vi "PrefDialog.vi"(8 "error in (no error)":errorcluster, 11 "MyPluginsBase in":refnum<class "ChromaAcLoad.lvclass">) -> (0 "error out":errorcluster, 1 "Save As":bool, 2 "Changed":bool, 3 "MyPluginsBase out":refnum<class "ChromaAcLoad.lvclass">)   [LabVIEW 2018, in "AcPwrPlugins.lvlib" / "ChromaAcLoad.lvclass"]
doc: "This VI opens up the modal preference dialog window and allows a user to configure the dialog with a new configuration or the existing configuration that was previously saved to file. The user can also chose to save the new configuration to the existing file location with the save boolean or a new file location by using the save as boolean."
uses:
  ChromaAcLoad.lvclass
  C:/Program Files (x86)/National Instruments/LabVIEW 2018/user.lib/NIST/BaseClasses/BasePlugin_class/BasePlugin.lvclass
  C:/Projects/ICDAS - Local tetsing/NistPluggableModules/AcPwr/AcPwrPlugins/AcPwrBaseClass/AcPwrBase.lvclass
  TypeDefs/Device(s)Settings.ctl
  TypeDefs/ConfigMode.ctl
  AcPwrBaseClass/TypeDefs/BaseMeasurements.ctl
  TypeDefs/MeasurementType.ctl
  TypeDefs/Measurements.ctl
  <userlib>/NIST/BaseClasses/BasePlugin_class/BasePlugin.lvclass/BasePlugin.ctl
  AcPwrBaseClass/AcPwrBase.lvclass/AcPwrBase.ctl
  <userlib>/NIST/BaseClasses/BasePlugin_class/Accessors/Read PluginIniFilePath.vi
  AcPwrBaseClass/Accessors/Read BaseConfig.vi
  AcPwrBaseClass/Accessors/Read BaseMeasurements.vi
  <userlib>/NIST/BaseClasses/BasePlugin_class/Accessors/Write PluginIniFilePath.vi
  <vilib>/Utility/config.llb/NI_LVConfig.lvlib
  AcPwrBaseClass/AcPwrBase.lvclass
panel:
  in  "Measurements":T1 caption="Measurements*"
  in  "BaseMeasurements":T3 {"NHRGridSim Phase" items=["All", "A Phase", "B Phase", "C Phase"]; "NHRDC Measurement Type" items=["Voltage"=1, "Positive Peak Voltage"=2, "Positive Peak Voltage Last Fetch"=4, "Negative Peak Voltage"=8, "Negative Peak Voltage Last Fetch"=16, "Current"=32, "Positive Peak Current"=64, "Positive Peak Current Last Fetch"=128, "Negative Peak Current"=256, "Negative Peak Current Last Fetch"=512, "Power"=1024, "Positive Peak Power"=2048, "Positive Peak Power Last Fetch"=4096, "Negative Peak Power"=8192, "Negative Peak Power Last Fetch"=16384, "Timestamp"=32768, "Charge Time"=65536, "Discharge Time"=131072, "Amp Hour"=262144, "Amp Hour Time"=524288, "Amp Hour Charge"=1048576, "Amp Hour Discharge"=2097152, "Kilo Watt Hour"=4194304, "Kilo Watt Hour Time"=8388608, "Kilo Watt Hour Charge"=16777216, "Kilo Watt Hour Discharge"=33554432, "UUT Temperature"=67108864]; "NHRDC Fetch Method" items=["Aperture", "Immediate"]}
  in  "Disable Controls based on Configuration Mode?":bool
  in  "Device(s)Settings":T4 {"Phases"."Phase Select" items=["Phase ALL", "Phase A", "Phase B", "Phase C"]; "Phases"."Slew Rate"."Fall Slew Rate (A/ms)" min=4 max=600 step=1; "Phases"."Slew Rate"."Rise Slew Rate (A/ms)" min=4 max=600 step=1}
  in  "btnSaveAs":bool
  in  "Measurement RefreshTime (ms)":u32
  in  "btnSave":bool
  in  "btnCancel":bool
  # "*Please ensure that Voltage and Current are selected as the 1st and 2nd Measurement variables, respectively, to correctly plot Voltage vs Current in the visualization VI."
  # "AC is compatible with: CC, CR, CP, RLC, RLC CP, and Inrush\n\nDC is compatible with: CC, CR, CP, CV, and Rectified"
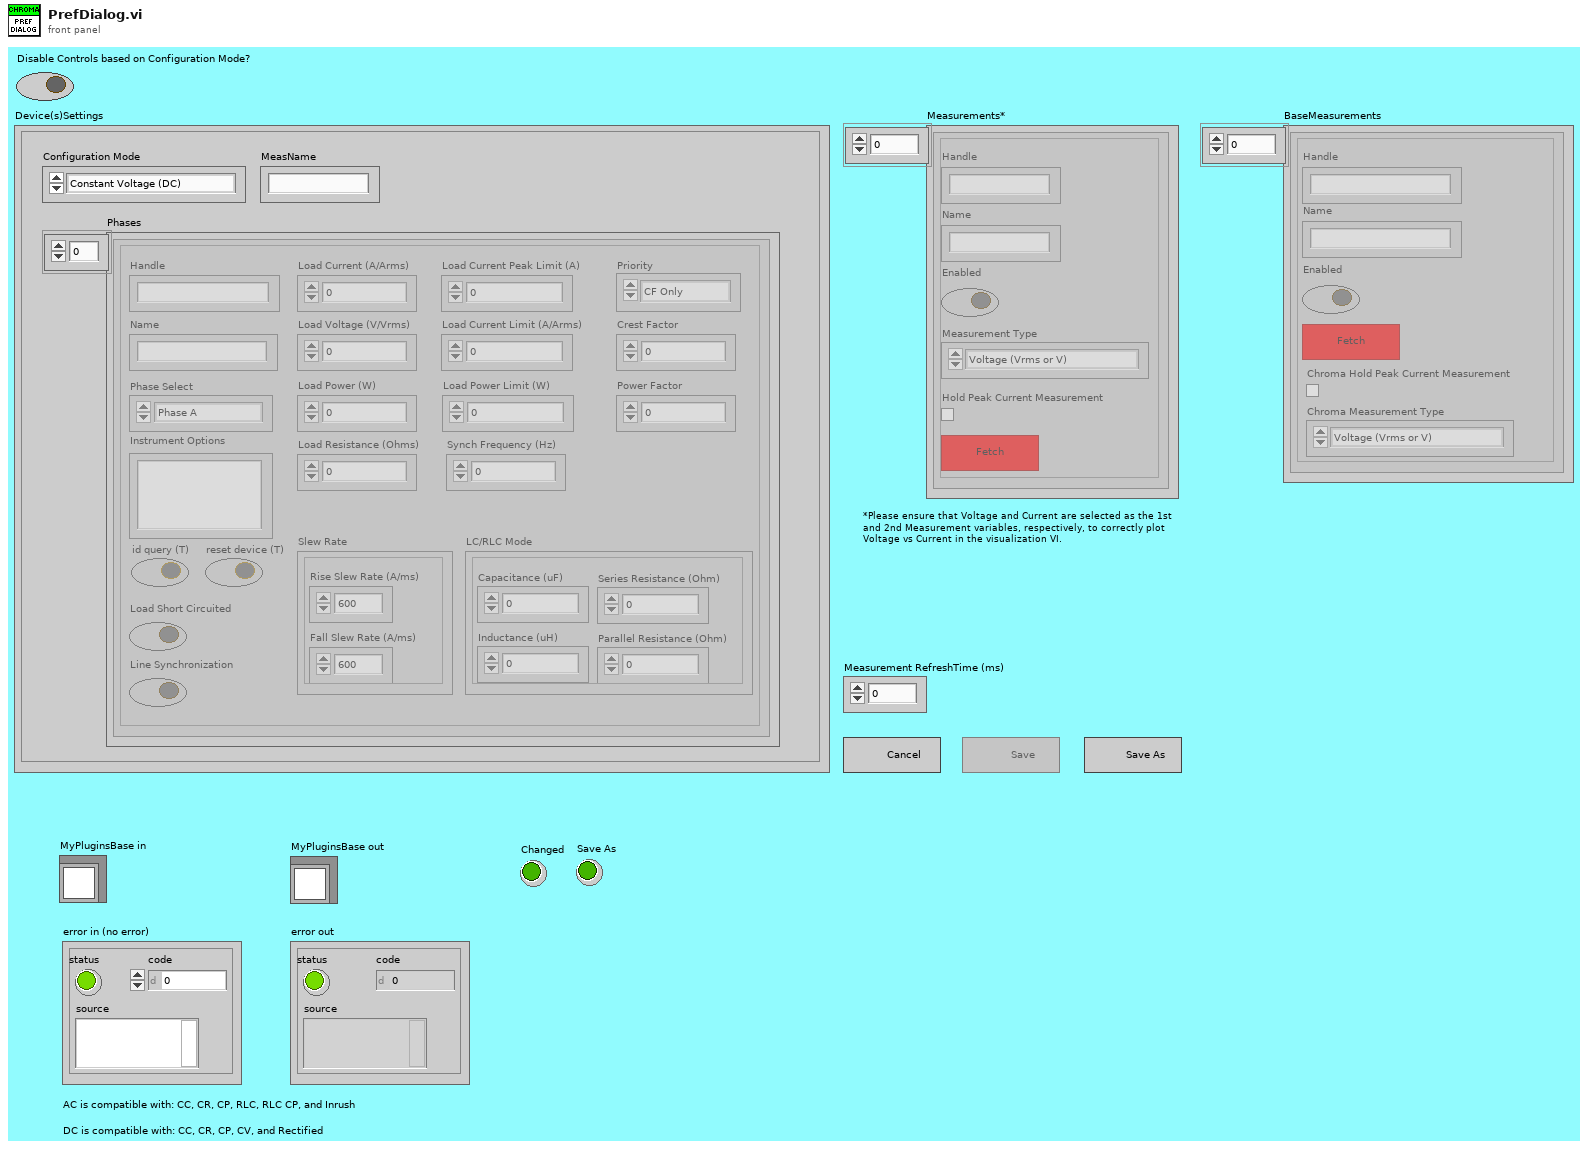
[diagram p1: front panel]
types:
  T1 = typedef "AcPwrPlugins.lvlib/ChromaAcLoad.lvclass/Measurements.ctl" = cluster{"Handle":string, "Name":string, "Enabled":bool, "Measurement Value":dbl, "Hold Peak Current Measurement":bool, "btnMeasFetch":bool, "ProtectionStatusString":string, "Measurement Type":T2}[]
  T2 = typedef "AcPwrPlugins.lvlib/ChromaAcLoad.lvclass/MeasurementType.ctl" = enum16{"Voltage (Vrms or V)", "Current (Arms or A)", "Power (W)", "Peak Voltage (V)", "Peak Current (A)", "Peak Power (W)", "Frequency (Hz)", "Resistance (Ohms)", "Voltage Overshoot (V)", "Positive Peak Current (A)", "Voltage Undershoot (V)", "Negative Peak Current (A)", "Apparent Power (VA)", "Reacitive Power (VAR)", "Voltage THD", "Power Factor", "Current's Crest Factor"}
  T3 = typedef "AcPwrPlugins.lvlib/AcPwrBase.lvclass/BaseMeasurements.ctl" = cluster{"Handle":string, "Name":string, "Enabled":bool, "Measurement Value":dbl, "btnMeasFetch":bool, "Chroma Hold Peak Current Measurement":bool, "Chroma Measurement Type":T2, "Chroma Protection Status String":string, "NHRDC Fetch Method":i32, "NHRDC Fetch Time (s)":sgl, "NHRDC Measurement Type":i32, "NHRGridSim Measurement Type ":enum16{"Average Current", "Max Current", "Min Current", "Average Voltage", "Max Voltage", "Min Voltage", "Average True Power", "Max True Power", "Min True Power", "Average Apparent Power", "Max Apparent Power", "Min Apparent Power", "Power Factor", "Crest Factor"}, "NHRGridSim Phase ":i32, "PPS Measurement Type ":enum16{"Voltage RMS L-N", "Voltage RMS L-L", "Frequency", "Current RMS", "Current Peak", "Crest Factor", "Power Factor", "Power VA", "Real Power"}, "PPS Channel Name":enum16{"A", "B", "C"}}[]
  T4 = typedef "AcPwrPlugins.lvlib/ChromaAcLoad.lvclass/Device(s)Settings.ctl" = cluster{"Configuration Mode":T5, "Phases":cluster{"Handle":string, "Name":string, "Phase Select":i32, "Instrument Options":string, "id query (T)":bool, "reset device (T)":bool, "Load Short Circuited":bool, "Line Synchronization":bool, "Load Current (A/Arms)":dbl, "Load Voltage (V/Vrms)":dbl, "Load Power (W)":dbl, "Load Resistance (Ohms)":dbl, "Load Current Peak Limit (A)":dbl, "Load Current Limit (A/Arms)":dbl, "Load Power Limit (W)":dbl, "Synch Frequency (Hz)":dbl, "Priority":enum16{"CF Only", "PF Only", "Both (CF)", "Both (PF)"}, "Crest Factor":dbl, "Power Factor":dbl, "Slew Rate":cluster{"Rise Slew Rate (A/ms)":i32, "Fall Slew Rate (A/ms)":i32}, "LC/RLC Mode":cluster{"Capacitance (uF)":i32, "Inductance (uH)":i32, "Series Resistance (Ohm)":dbl, "Parallel Resistance (Ohm)":dbl}, "Timing":cluster{"TimingOn":enum16{""}, "Hours":u32, "Minutes":u32, "Seconds":dbl, "CutoffVoltage":dbl}, "Connected":bool}[], "MeasName":string}
  T5 = typedef "ConfigMode.ctl" = enum16{"Constant Voltage (DC)", "Constant Power (DC)", "Constant Power (AC)", "Constant Current (DC)", "Constant Current (AC)", "Constant Resistance (DC)", "Constant Resistance (AC)", "Rectified Mode (DC)", "Inrush (AC)", "RLC CP (AC)", "RLC (AC)"}
  T6 = enum32{"Invalid", "Default", "Floating", "Floating/Auto-Hide", "Modal"}
  T7 = enum32{"Invalid", "Standard", "Closed", "Hidden", "Minimized", "Maximized"}
  T8 = enum8{"Enabled", "Disabled", "Disabled and Grayed Out"}
  T9 = cluster{"Handle":string, "Name":string, "Phase Select":i32, "Instrument Options":string, "id query (T)":bool, "reset device (T)":bool, "Load Short Circuited":bool, "Line Synchronization":bool, "Load Current (A/Arms)":dbl, "Load Voltage (V/Vrms)":dbl, "Load Power (W)":dbl, "Load Resistance (Ohms)":dbl, "Load Current Peak Limit (A)":dbl, "Load Current Limit (A/Arms)":dbl, "Load Power Limit (W)":dbl, "Synch Frequency (Hz)":dbl, "Priority":enum16{"CF Only", "PF Only", "Both (CF)", "Both (PF)"}, "Crest Factor":dbl, "Power Factor":dbl, "Slew Rate":cluster{"Rise Slew Rate (A/ms)":i32, "Fall Slew Rate (A/ms)":i32}, "LC/RLC Mode":cluster{"Capacitance (uF)":i32, "Inductance (uH)":i32, "Series Resistance (Ohm)":dbl, "Parallel Resistance (Ohm)":dbl}, "Timing":cluster{"TimingOn":enum16{""}, "Hours":u32, "Minutes":u32, "Seconds":dbl, "CutoffVoltage":dbl}, "Connected":bool}[]
  T10 = cluster{"Handle":string, "Name":string, "Phase Select":i32, "Instrument Options":string, "id query (T)":bool, "reset device (T)":bool, "Load Short Circuited":bool, "Line Synchronization":bool, "Load Current (A/Arms)":dbl, "Load Voltage (V/Vrms)":dbl, "Load Power (W)":dbl, "Load Resistance (Ohms)":dbl, "Load Current Peak Limit (A)":dbl, "Load Current Limit (A/Arms)":dbl, "Load Power Limit (W)":dbl, "Synch Frequency (Hz)":dbl, "Priority":enum16{"CF Only", "PF Only", "Both (CF)", "Both (PF)"}, "Crest Factor":dbl, "Power Factor":dbl, "Slew Rate":cluster{"Rise Slew Rate (A/ms)":i32, "Fall Slew Rate (A/ms)":i32}, "LC/RLC Mode":cluster{"Capacitance (uF)":i32, "Inductance (uH)":i32, "Series Resistance (Ohm)":dbl, "Parallel Resistance (Ohm)":dbl}, "Timing":cluster{"TimingOn":enum16{""}, "Hours":u32, "Minutes":u32, "Seconds":dbl, "CutoffVoltage":dbl}, "Connected":bool}
  T11 = typedef "AcPwrPlugins.lvlib/AcPwrBase.lvclass/BaseConfig.ctl" = cluster{"Frequency":dbl, "FrequencyRange":dbl[], "Phases":T12[], "Name":string, "PluginConfigVariant":variant, "PluginMeasVariant":variant}
  T12 = typedef "AcPwrPlugins.lvlib/AcPwrBase.lvclass/Phase.ctl" = cluster{"Name":string, "Enabled":bool, "VoltageLevel":dbl, "Handle":string, "VoltageRange":dbl[], "Connected":bool, "CurrentLimit":dbl, "Waveform":string}
  T13 = typedef "NI_LVConfig.lvlib/Config Data RefNum.ctl" = refnum<k1>
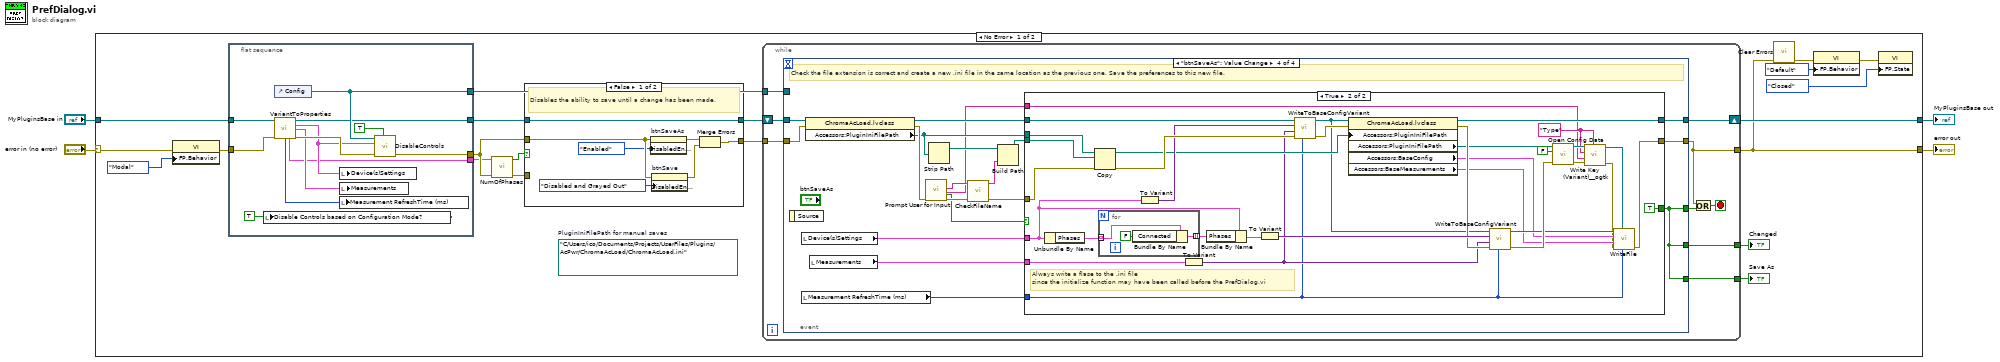
[diagram p0: block diagram]
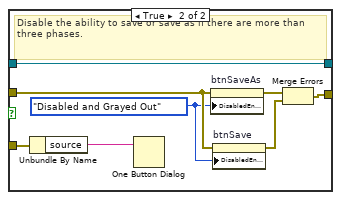
[diagram p2: hidden frame]
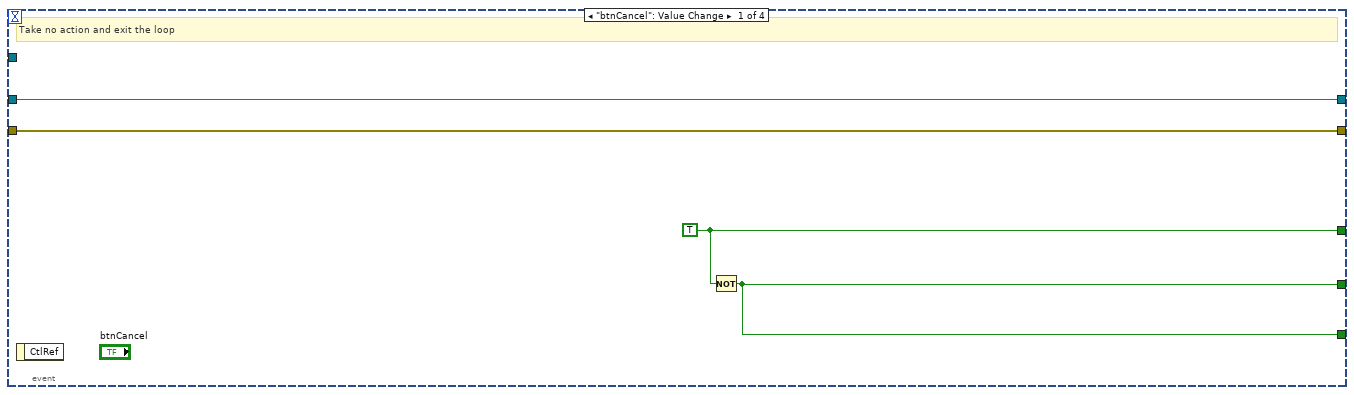
[diagram p3: hidden frame]
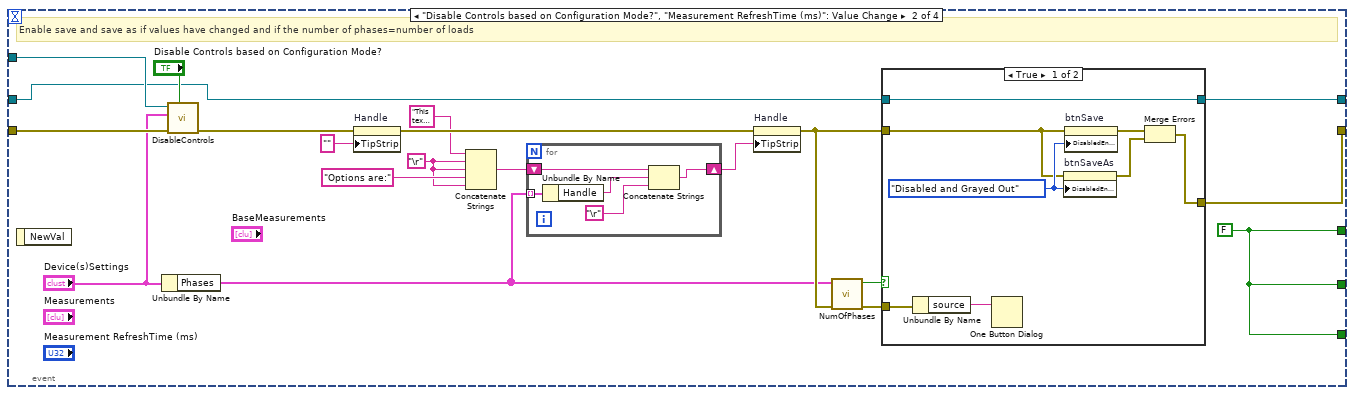
[diagram p4: hidden frame]
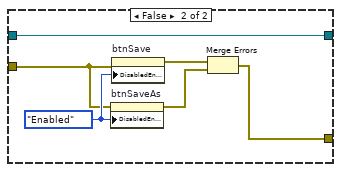
[diagram p5: hidden frame]
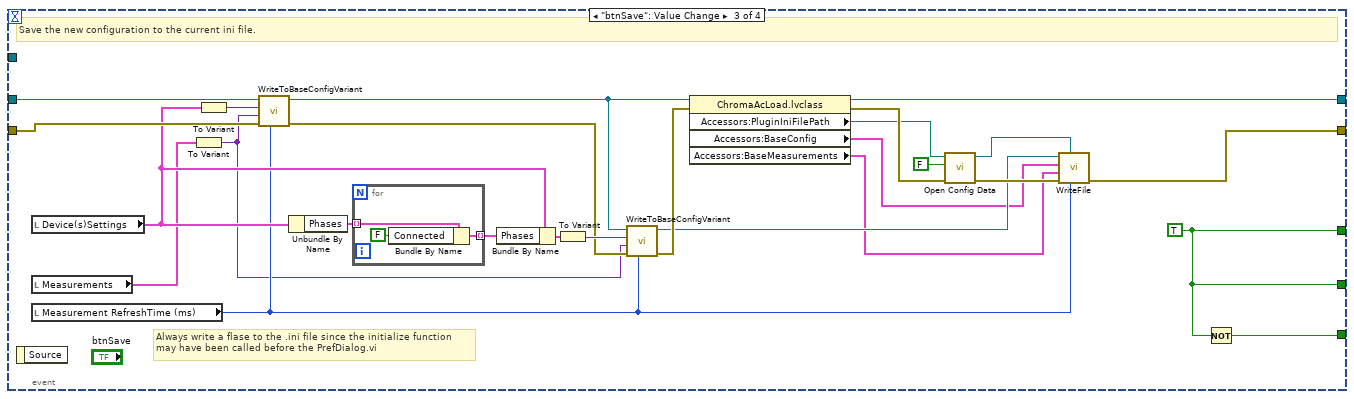
[diagram p6: hidden frame]
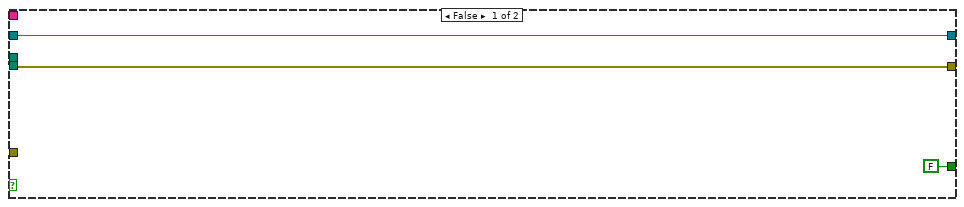
[diagram p7: hidden frame]
diagram:
  n1 = case shown="No Error" "error in (no error)" {
    selector: "error in (no error)" -> [w18 w191]
    tunnel: [w24 w192] -> w4
    tunnel: [w5 w191] -> w3
    tunnel: "MyPluginsBase in" -> [w20 w192]
    frame No Error {
      (unwired) path "C:/Users/ico/Documents/Projects/UserFiles/Plugins/AcPwr/ChromaAcLoad/ChromaAcLoad.ini"  # PluginIniFilePath for manual saves
      n2 = property class="VI"(error in=w18, "FP.Behavior"=T6."Modal" ("Front Panel Window:Behavior")) -> (error out=w16:errorcluster)  [unwired: 1 in, 1 out]
      n3 = flat-sequence {
        tunnel: w20 -> [w36]
        tunnel: [w28] -> w8
        tunnel: [w34] -> w10
        tunnel: w16 -> [w35]
        tunnel: [w25] -> w9
        tunnel: [w31] -> w11
        frame #0 {
          n4 = local write "Disable Controls based on Configuration Mode?"(TRUE ("Enable Disabling of Controls based on Configuration Mode")) -> ()
          n5 = control-ref of="Config"() -> (w31:refnum<vi>)
          n6 = call "VariantToProperties.vi"("ChromaAcLoad"=w36, "error in (no error)"=w35) -> ("ChromaAcLoad"=w28:refnum<class "ChromaAcLoad.lvclass">, "Device Properties"=w29:T4, "Meas"=w26:T1, "Measurement Refresh Time (ms)"=w27:u32, "Phases"=w25:T9, "error out"=w30:errorcluster)  [unwired: 7 in, 1 out]
          n7 = local write "Measurement RefreshTime (ms)"(w27) -> ()
          n8 = local write "Device(s)Settings"(w29) -> ()
          n9 = local write "Measurements"(w26) -> ()
          n10 = call "DisableControls.vi"("Enable (T)"=TRUE ("Enable"), "error in (no error)"=w30, "Device Properties In"=w29, "Cluster"=w31) -> ("Error Out"=w34:errorcluster)  [unwired: 6 in, 1 out]
        }
      }
      n11 = call "NumOfPhases.vi"("Error In"=w10, "Phases"=w9) -> ("Error Out"=w12:errorcluster, "NumberOfPhases>3"=w13:bool)  [unwired: 8 in]
      n12 = case shown="False" w13 {
        tunnel: w10 -> [w43 w51]
        tunnel: [w39 w47] -> w14
        tunnel: w12 -> [_ w45]
        tunnel: w8 -> [w37 w44]
        tunnel: [w37 w44] -> w7
        frame False {
          # "Disables the ability to save until a change has been made."
          n13 = property on="btnSaveAs" class="Bool"(error in=w43, "DisabledEnum"=T8."Enabled" ("Disabled")) -> (error out=w40:errorcluster)  [unwired: 1 in, 1 out]
          n14 = property on="btnSave" class="Bool"(error in=w43, "DisabledEnum"=T8."Disabled and Grayed Out" ("Disabled")) -> (error out=w41:errorcluster)  [unwired: 1 in, 1 out]
          n15 = Merge Errors(w40, w41) -> (w39:errorcluster)
        }
        frame True {
          w50 = T8."Disabled and Grayed Out" ("Disabled")
          # "Disable the ability to save or save as if there are more than three phases."
          n16 = Unbundle By Name(w45) -> ("source"=w46:string)
          n17 = One Button Dialog(message=w46) -> ()  [unwired: 1 in, 1 out]
          n18 = property on="btnSaveAs" class="Bool"(error in=w51, "DisabledEnum"=w50) -> (error out=w48:errorcluster)  [unwired: 1 in, 1 out]
          n19 = property on="btnSave" class="Bool"(error in=w51, "DisabledEnum"=w50) -> (error out=w49:errorcluster)  [unwired: 1 in, 1 out]
          n20 = Merge Errors(w48, w49) -> (w47:errorcluster)
        }
      }
      n21 = while {
        shift-right: [w59] -> w24
        shift-left: w7 -> [w60]
        tunnel: w14 -> [w58]
        tunnel: [w54] -> w5
        tunnel: [w57] -> w19
        tunnel: [w56] -> w15
        tunnel: w11 -> [w52]
        stop <- w55 stop-if-true
        n22 = event shown="[3] \"btnSaveAs\": Value Change" {
          selector: _ -> [_ _ _ _]
          dyn-events: _ -> [_ _ _ _]
          timeout: _ -> [_ _ _ _]
          tunnel: w60 -> [w64 w66 w119 w150]
          tunnel: [w62 w83 w127 w151] -> w53
          tunnel: [w64 w82 w111 w145] -> w59
          tunnel: w58 -> [w63 w77 w118 w149]
          tunnel: [w63 w84 w120 w148] -> w54
          tunnel: [w61 w83 w127 w151] -> w57
          tunnel: [w61 w83 w126 w151] -> w56
          tunnel: w52 -> [_ w69 _ _]
          event "btnCancel": Value Change {
            w62 = TRUE
            # "Take no action and exit the loop"
            n23 = event-data() -> ()  [unwired: 1 in, 1 out]
            n24 = Not(x=w62) -> (.not. x?=w61:bool)
          }
          event "Disable Controls based on Configuration Mode?", "Measurement RefreshTime (ms)": Value Change {
            w72 = "\r"
            w83 = FALSE
            # "Enable save and save as if values have changed and if the number of phases=number of loads"
            n25 = event-data() -> ()  [unwired: 1 in, 1 out]
            n26 = Unbundle By Name("Device(s)Settings") -> ("Phases"=w65:T9)
            n27 = call "DisableControls.vi"("Enable (T)"="Disable Controls based on Configuration Mode?", "error in (no error)"=w77, "Device Properties In"="Device(s)Settings", "Cluster"=w69) -> ("Error Out"=w67:errorcluster)  [unwired: 6 in, 1 out]
            n28 = property on="Handle" class="Str"(error in=w67, "TipStrip"="" ("Tip Strip")) -> (error out=w79:errorcluster)  [unwired: 1 in, 1 out]
            n29 = Concatenate Strings("This text in this handle of the instrument and entered in the  \nhandle control in the Phases array EXACTLY, lest the attempt \nto interact with the instrument will fail.", w72, w72, "Options are:" ("Handle"), w72) -> (w78:string)
            n30 = for {
              shift-right: [w89] -> w80
              shift-left: w78 -> [w88]
              tunnel: w65 -> [w87] mode=indexing
              n31 = Unbundle By Name(w87) -> ("Handle"=w86:string)
              n32 = Concatenate Strings(w88, w86, "\r") -> (w89:string)
            }
            n33 = property on="Handle" class="Str"(error in=w79, "TipStrip"=w80) -> (error out=w68:errorcluster)  [unwired: 1 in, 1 out]
            n34 = call "NumOfPhases.vi"("Error In"=w68, "Phases"=w65) -> ("Error Out"=w81:errorcluster, "NumberOfPhases>3"=w70:bool)  [unwired: 8 in]
            n35 = case shown="True" w70 {
              tunnel: w68 -> [w94 w100]
              tunnel: [w93 w99] -> w84
              tunnel: w66 -> [w92 w98]
              tunnel: [w92 w98] -> w82
              tunnel: w81 -> [w90 _]
              frame True {
                w95 = T8."Disabled and Grayed Out" ("Disabled")
                n36 = Unbundle By Name(w90) -> ("source"=w91:string)
                n37 = One Button Dialog(message=w91) -> ()  [unwired: 1 in, 1 out]
                n38 = property on="btnSaveAs" class="Bool"(error in=w94, "DisabledEnum"=w95) -> (error out=w97:errorcluster)  [unwired: 1 in, 1 out]
                n39 = property on="btnSave" class="Bool"(error in=w94, "DisabledEnum"=w95) -> (error out=w96:errorcluster)  [unwired: 1 in, 1 out]
                n40 = Merge Errors(w96, w97) -> (w93:errorcluster)
              }
              frame False {
                w101 = T8."Enabled" ("Disabled")
                n41 = property on="btnSaveAs" class="Bool"(error in=w100, "DisabledEnum"=w101) -> (error out=w103:errorcluster)  [unwired: 1 in, 1 out]
                n42 = property on="btnSave" class="Bool"(error in=w100, "DisabledEnum"=w101) -> (error out=w102:errorcluster)  [unwired: 1 in, 1 out]
                n43 = Merge Errors(w102, w103) -> (w99:errorcluster)
              }
            }
          }
          event "btnSave": Value Change {
            w127 = TRUE
            # "Always write a flase to the .ini file since the initialize function\nmay have been called before the PrefDialog.vi"
            # "Save the new configuration to the current ini file."
            n44 = event-data() -> ()  [unwired: 1 in, 1 out]
            n45 = local read "Device(s)Settings"() -> (w109:T4)
            n46 = local read "Measurements"() -> (w105:T1)
            n47 = local read "Measurement RefreshTime (ms)"() -> (w107:u32)
            n48 = To Variant(anything=w105) -> (Variant=w106:variant)
            n49 = To Variant(anything=w109) -> (Variant=w117:variant)
            n50 = call "WriteToBaseConfigVariant.vi"("Measurement Refresh Time (ms)"=w107, "error in (no error)"=w118, "Meas"=w106, "Config"=w117, "ChromaAcLoad in"=w119) -> ("error out"=w113:errorcluster, "ChromaAcLoad out"=w114:refnum<class "ChromaAcLoad.lvclass">)  [unwired: 5 in]
            n51 = Unbundle By Name(w109) -> ("Phases"=w124:T9)
            n52 = for {
              tunnel: w124 -> [w131] mode=indexing
              tunnel: [w132] -> w123 mode=indexing
              n53 = Bundle By Name(cluster=w131, "Connected"=FALSE) -> (w132:T10)
            }
            n54 = Bundle By Name(cluster=w109, "Phases"=w123) -> (w115:T4)
            n55 = To Variant(anything=w115) -> (Variant=w116:variant)
            n56 = call "WriteToBaseConfigVariant.vi"("Measurement Refresh Time (ms)"=w107, "error in (no error)"=w113, "Meas"=w106, "Config"=w116, "ChromaAcLoad in"=w114) -> ("error out"=w112:errorcluster, "ChromaAcLoad out"=w110:refnum<class "ChromaAcLoad.lvclass">)  [unwired: 5 in]
            n57 = property class="ChromaAcLoad.lvclass"(reference=w114, error in=w112) -> (reference out=w111:refnum<class "ChromaAcLoad.lvclass">, error out=w129:errorcluster, "Accessors:PluginIniFilePath"=w125:path, "Accessors:BaseConfig"=w108:T11, "Accessors:BaseMeasurements"=w104:T3)
            n58 = call <vilib>:"Open Config Data.vi"("error in (no error)"=w129, "create file if necessary (T)"=FALSE, "configuration file path"=w125) -> ("error out"=w122:errorcluster, "refnum"=w121:T13)  [unwired: 6 in, 1 out]
            n59 = call-dynamic "WriteFile.vi"("Measurement RefreshTime (ms)"=w107, "Refnum in"=w121, "error in (no error)"=w122, "BaseMeasurements"=w104, "BaseConfiguration"=w108, "ChromaAcLoad in"=w110) -> ("error out"=w120:errorcluster)  [unwired: 4 in, 1 out]
            n60 = Not(x=w127) -> (.not. x?=w126:bool)
          }
          event "btnSaveAs": Value Change {
            # "Check the file extension is correct and create a new .ini file in the same location as the previous one. Save the preferences to this new file."
            n61 = event-data() -> ()  [unwired: 1 in, 1 out]
            n62 = local read "Device(s)Settings"() -> (w146:T4)
            n63 = local read "Measurement RefreshTime (ms)"() -> (w143:u32)
            n64 = property class="ChromaAcLoad.lvclass"(reference=w150, error in=w149) -> (reference out=w147:refnum<class "ChromaAcLoad.lvclass">, error out=w142:errorcluster, "Accessors:PluginIniFilePath"=w137:path)
            n65 = local read "Measurements"() -> (w144:T1)
            n66 = call "Prompt User for Input"("error in (no error)"=w142) -> ("File Name"=w140:string, "PluginType"=w133:string, "OK"=w134:bool, "error out"=w141:errorcluster)  [unwired: 15 in]
            n67 = Strip Path(path=w137) -> (stripped path=w139:path)  [unwired: 1 out]
            n68 = call "CheckFileName.vi"("Error In"=w141, "File Name in"=w140) -> ("Error Out"=w135:errorcluster, "File Name out"=w138:string)  [unwired: 8 in]
            n69 = Build Path(base path=w139, name or relative path=w138) -> (appended path=w136:path)
            n70 = case shown="True" w134 {
              tunnel: [FALSE TRUE] -> w151
              tunnel: w137 -> [_ w185]
              tunnel: [w153 w182] -> w148
              tunnel: w147 -> [w154 w181]
              tunnel: w146 -> [_ w177]
              tunnel: [w154 w161] -> w145
              tunnel: w144 -> [_ w167]
              tunnel: w143 -> [_ w165]
              tunnel: w136 -> [_ w164]
              tunnel: w135 -> [w153 w163]
              tunnel: w133 -> [_ w157]
              frame False {
              }
              frame True {
                w158 = "Type" ("section")
                # "Always write a flase to the .ini file\nsince the initialize function may have been called before the PrefDialog.vi"
                n71 = Unbundle By Name(w177) -> ("Phases"=w184:T9)
                n72 = Copy(8:w163, 10:w164, 11:w185) -> (0:w179:errorcluster, 3:w171:path)  [unwired: 2 in, 1 out]
                n73 = for {
                  tunnel: w184 -> [w188] mode=indexing
                  tunnel: [w190] -> w183 mode=indexing
                  n74 = Bundle By Name(cluster=w188, "Connected"=FALSE) -> (w190:T10)
                }
                n75 = To Variant(anything=w177) -> (Variant=w178:variant)
                n76 = To Variant(anything=w167) -> (Variant=w166:variant)
                n77 = Bundle By Name(cluster=w177, "Phases"=w183) -> (w176:T4)
                n78 = To Variant(anything=w176) -> (Variant=w175:variant)
                n79 = call "WriteToBaseConfigVariant.vi"("Measurement Refresh Time (ms)"=w165, "error in (no error)"=w179, "Meas"=w166, "Config"=w178, "ChromaAcLoad in"=w181) -> ("error out"=w180:errorcluster, "ChromaAcLoad out"=w162:refnum<class "ChromaAcLoad.lvclass">)  [unwired: 5 in]
                n80 = property class="ChromaAcLoad.lvclass"(reference=w162, error in=w180, "Accessors:PluginIniFilePath"=w171) -> (reference out=w161:refnum<class "ChromaAcLoad.lvclass">, error out=w174:errorcluster, "Accessors:PluginIniFilePath"=w170:path, "Accessors:BaseConfig"=w169:T11, "Accessors:BaseMeasurements"=w168:T3)
                n81 = call "WriteToBaseConfigVariant.vi"("Measurement Refresh Time (ms)"=w165, "error in (no error)"=w174, "Meas"=w166, "Config"=w175, "ChromaAcLoad in"=w162) -> ("error out"=w173:errorcluster, "ChromaAcLoad out"=w172:refnum<class "ChromaAcLoad.lvclass">)  [unwired: 5 in]
                n82 = call <vilib>:"Open Config Data.vi"("error in (no error)"=w173, "create file if necessary (T)"=FALSE, "configuration file path"=w170) -> ("error out"=w160:errorcluster, "refnum"=w159:T13)  [unwired: 6 in, 1 out]
                n83 = call <userlib>:"Write Key (Variant)__ogtk.vi"("section"=w158, "error in (no error)"=w160, "key-value"=w157, "key (optional)"=w158, "refnum"=w159) -> ("error out"=w156:errorcluster, "refnum out"=w155:T13)  [unwired: 5 in]
                n84 = call-dynamic "WriteFile.vi"("Measurement RefreshTime (ms)"=w165, "Refnum in"=w155, "error in (no error)"=w156, "BaseMeasurements"=w168, "BaseConfiguration"=w169, "ChromaAcLoad in"=w172) -> ("error out"=w182:errorcluster)  [unwired: 4 in, 1 out]
              }
            }
          }
        }
        n85 = Or(x=w54, y=w53) -> (x .or. y?=w55:bool)
      }
      "Changed" <- w19
      "Save As" <- w15
      n86 = call <vilib>:"Clear Errors.vi"("error in (no error)"=w5) -> ("error out"=w6:errorcluster)  [unwired: 5 in, 1 out]
      n87 = property class="VI"(error in=w6, "FP.Behavior"=T6."Default" ("Front Panel Window:Behavior")) -> (error out=w23:errorcluster)  [unwired: 1 in, 1 out]
      n88 = property class="VI"(error in=w23, "FP.State"=T7."Closed" ("Front Panel Window:State")) -> ()  [unwired: 1 in, 2 out]
    }
    frame Error {
    }
  }
  "error out" <- w3
  "MyPluginsBase out" <- w4
